vi "Update Front Panel.vi"(9 "Table Data":variant, 11 "MediatorBusMonitor In":refnum<class "IMediatorBusMonitor.lvclass">) -> (3 "MediatorBusMonitor Out":refnum<class "IMediatorBusMonitor.lvclass">)   [LabVIEW 2015]
uses:
  MediatorBusMonitor/IMediatorBusMonitor.lvclass
panel:
  out "error out":errorcluster
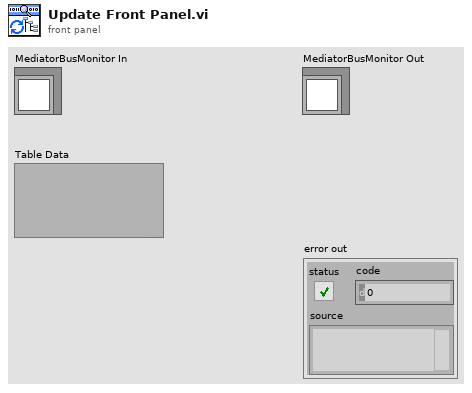
[diagram p1: front panel]
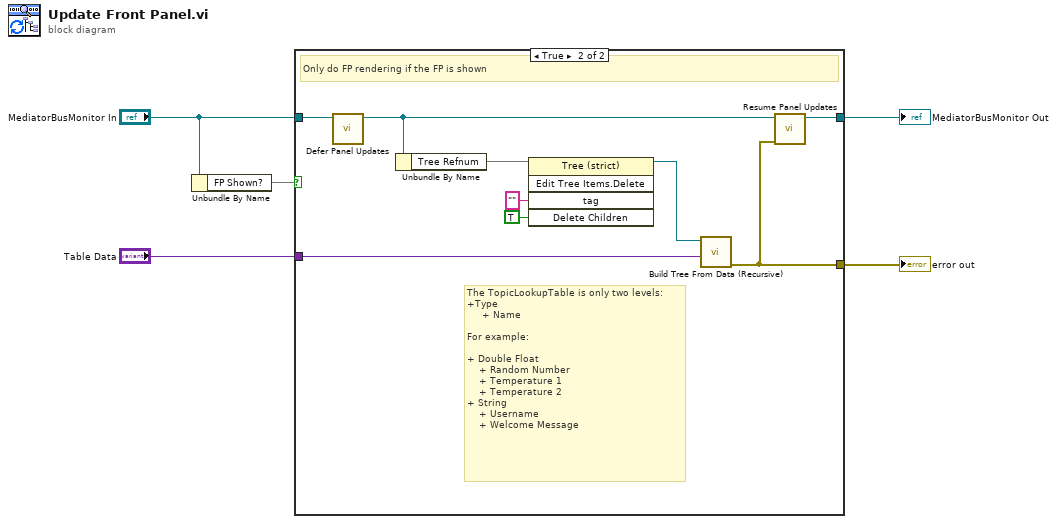
[diagram p0: block diagram]
diagram:
  n1 = Unbundle By Name("MediatorBusMonitor In") -> ("FP Shown?"=w1)
  n2 = case shown="True" w1 {
    tunnel: "MediatorBusMonitor In" -> [w6 w15]
    tunnel: "Table Data" -> [_ w14]
    tunnel: [w6 w8] -> w4
    tunnel: [_ w7] -> w3
    frame False {
    }
    frame True {
      # "The TopicLookupTable is only two levels:\n+Type\n     + Name\n\nFor example:\n\n+ Double Float\n    + Random Number\n    + Temperature 1\n    + Temperature 2\n+ String\n    + Username\n    + Welcome Message"
      # "Only do FP rendering if the FP is shown"
      n3 = call-dynamic "Defer Panel Updates.vi"("IViewable In"=w15) -> ("IViewable Out"=w9:refnum<class "IMediatorBusMonitor.lvclass">)  [unwired: 9 in, 1 out]
      n4 = Unbundle By Name(w9) -> ("Tree Refnum"=w13)
      n5 = invoke class="Tree (strict)" method="Edit Tree Items.Delete"(reference=w13, "tag"="" ("Tag"), "Delete Children"=TRUE ("Delete Children?")) -> (reference out=w12:refnum<vi>)  [unwired: 2 in, 4 out]
      n6 = call "Build Tree From Data (Recursive).vi"("Variant"=w14, "TreeControl Ref"=w12) -> ("error out"=w7:errorcluster)  [unwired: 7 in, 2 out]
      n7 = call-dynamic "Resume Panel Updates.vi"("error in (no error)"=w7, "IViewable In"=w9) -> ("IViewable Out"=w8:refnum<class "IMediatorBusMonitor.lvclass">)  [unwired: 8 in, 1 out]
    }
  }
  "MediatorBusMonitor Out" <- w4
  "error out" <- w3
